vi "Merge Error.vi"(10 "Error":errorcluster, 11 "TEMPLATE Actor in":refnum<class "TEMPLATE Actor.lvclass">) -> (3 "TEMPLATE Actor out":refnum<class "TEMPLATE Actor.lvclass">)   [LabVIEW 2020, in "_Template.lvlib" / "Templates.lvlib" / "TEMPLATE Actor.lvlib" / "TEMPLATE Actor.lvclass"]
uses:
  TEMPLATE Actor.lvclass
  TEMPLATE Actor.lvclass/TEMPLATE Actor.ctl
  jettl/jettl/Actor/Actor/Actor.lvclass
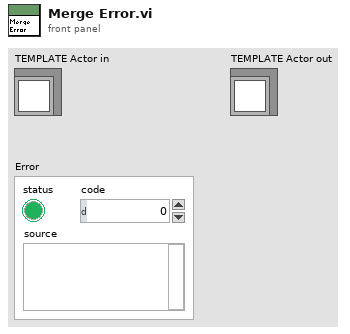
[diagram p1: front panel]
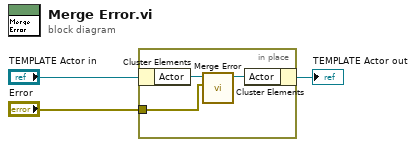
[diagram p0: block diagram]
diagram:
  n1 = in-place {
    in-place-border: "Error" -> [w4]
    n2 = in-place-cluster #1("TEMPLATE Actor in") -> ("Actor"=w6:refnum<class "Actor.lvclass">)
    n3 = call-dynamic "Merge Error.vi"("Error"=w4, "Actor in"=w6) -> ("Actor out"=w5:refnum<class "Actor.lvclass">)  [unwired: 9 in]
    n4 = in-place-cluster #1("Actor"=w5) -> (→"TEMPLATE Actor out":refnum<class "TEMPLATE Actor.lvclass">)
  }
